vi "Destroy Logger.vi"(8 "error in (no error)":errorcluster, 11 "Logger.Error in":refnum<class "Logger.Error.lvclass">) -> (0 "error out":errorcluster, 3 "Logger.Error out":refnum<class "Logger.Error.lvclass">)   [LabVIEW 2019, in "Logger.Error.lvclass"]
uses:
  Logger.Error.lvclass
  <userlib>/LevyLab/Logger/Logger.lvclass
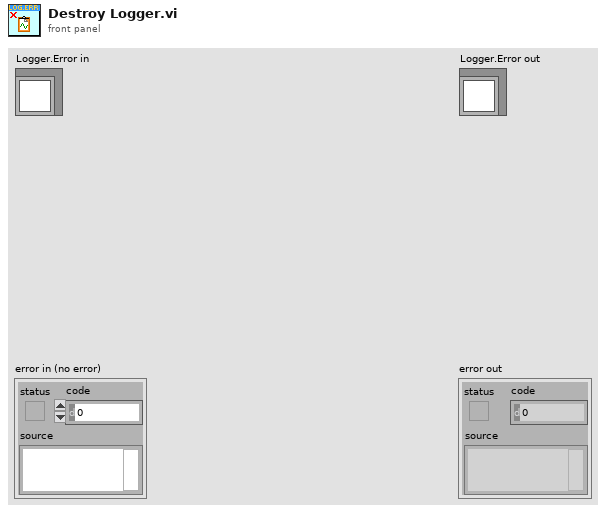
[diagram p1: front panel]
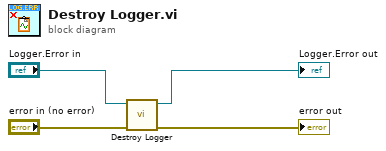
[diagram p0: block diagram]
diagram:
  n1 = call-parent "Destroy Logger.vi"("error in (no error)"="error in (no error)", "Logger in"="Logger.Error in") -> ("error out"=→"error out":errorcluster, "Logger out"=→"Logger.Error out":refnum<class "Logger.Error.lvclass">)  [unwired: 8 in]
